vi "Create Resources - FXP32 Address - FXP32 Data.vi"(0 "clip resources in":T1, 5 "address space size":u32, 7 "address space uid":u16) -> (4 "niInstr AXI4-Lite address space collection v1 FPGA out":refnum<class "niInstr AXI4-Lite Address Space Collection v1 FPGA.lvclass">)   [LabVIEW 2015, in "niInstr AXI4-Lite Address Space Collection v1 FPGA.lvclass"]
uses:
  <instrlib>/_niInstr/CLIP Adapters/v1/FPGA/AXI4-Lite/Address Space Collection/niInstr AXI4-Lite Address Space Collection v1 FPGA.lvclass
  <instrlib>/_niInstr/CLIP Adapters/v1/FPGA/AXI4-Lite/FXP32 Address - FXP32 Data/Public/CLIP Resources.ctl
  <instrlib>/_niInstr/CLIP Adapters/v1/FPGA/AXI4-Lite/Address Space Collection/niInstr AXI4-Lite Address Space Collection v1 FPGA.lvclass/niInstr AXI4-Lite Address Space Collection v1 FPGA.ctl
  <instrlib>/_niInstr/CLIP Adapters/v1/FPGA/AXI4-Lite/FXP32 Address - FXP32 Data/niInstr AXI4-Lite - FXP32 Address - FXP32 Data v1 FPGA.lvclass
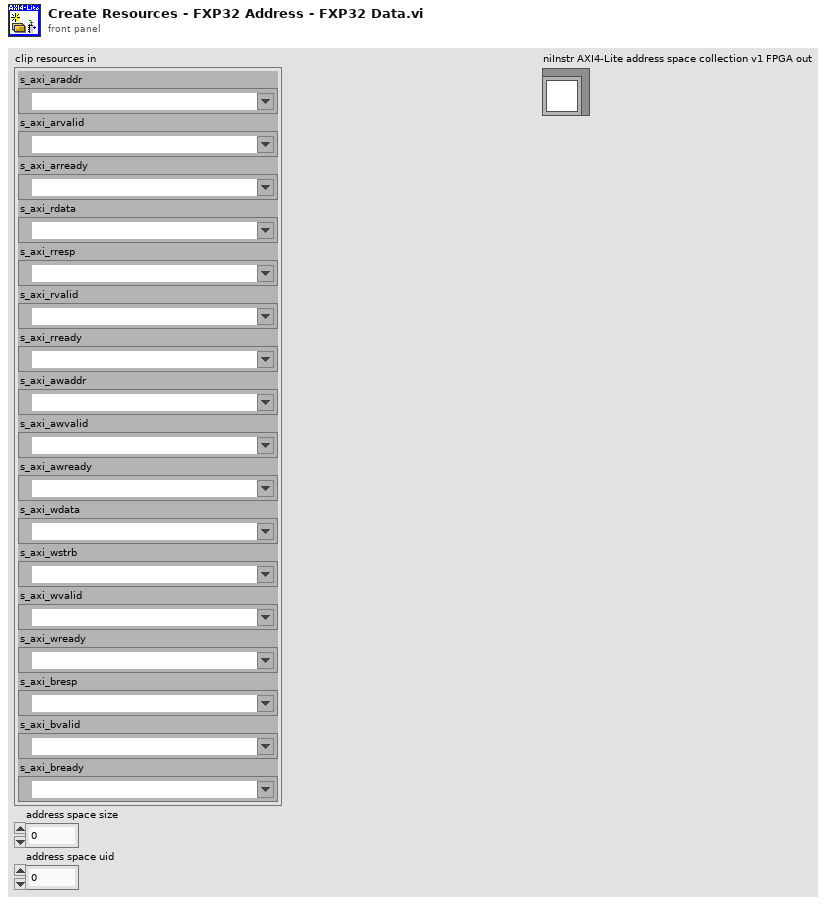
[diagram p1: front panel]
types:
  T1 = typedef "niInstr AXI4-Lite - FXP32 Address - FXP32 Data v1 FPGA.lvclass/CLIP Resources.ctl" = cluster{"s_axi_araddr":refnum<k21>, "s_axi_arvalid":refnum<k21>, "s_axi_arready":refnum<k21>, "s_axi_rdata":refnum<k21>, "s_axi_rresp":refnum<k21>, "s_axi_rvalid":refnum<k21>, "s_axi_rready":refnum<k21>, "s_axi_awaddr":refnum<k21>, "s_axi_awvalid":refnum<k21>, "s_axi_awready":refnum<k21>, "s_axi_wdata":refnum<k21>, "s_axi_wstrb":refnum<k21>, "s_axi_wvalid":refnum<k21>, "s_axi_wready":refnum<k21>, "s_axi_bresp":refnum<k21>, "s_axi_bvalid":refnum<k21>, "s_axi_bready":refnum<k21>}
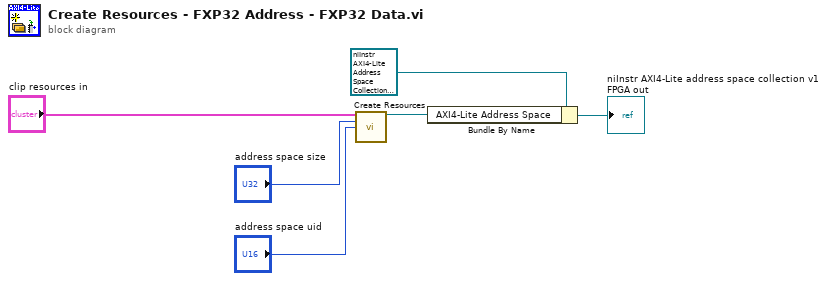
[diagram p0: block diagram]
diagram:
  n1 = call <instrlib>:"Create Resources.vi"("clip resources in"="clip resources in", "address space size"="address space size", "address space uid"="address space uid") -> ("niInstr AXI4-Lite - FXP32 address - fxp32 data v1 FPGA out"=w1:refnum<class "niInstr AXI4-Lite - FXP32 Address - FXP32 Data v1 FPGA.lvclass">)  [unwired: 12 in]
  n2 = Bundle By Name(cluster=refnum<class "niInstr AXI4-Lite Address Space Collection v1 FPGA.lvclass"> refnum ("AXI4-Lite Address Space Collection in"), "AXI4-Lite Address Space"=w1) -> (→"niInstr AXI4-Lite address space collection v1 FPGA out":refnum<class "niInstr AXI4-Lite Address Space Collection v1 FPGA.lvclass">)
